vi "R vs T measurement.vi"() -> ()   [LabVIEW 2017]
uses:
  <vilib>/Utility/file.llb/Read Delimited Spreadsheet (DBL).vi
  <vilib>/Utility/file.llb/Write Delimited Spreadsheet (DBL).vi
  <instrlib>/Lake Shore 336/Lake Shore 336.lvlib
panel:
  in  "Tab Control":enum32{"Controlls", "Graphs", "Diagnositcs"}(tab)
  in  "Source Meter address":refnum<visa-resource-name>="GPIB1::29::INSTR"
  out "Measured Resistance (Ohms)":dbl format="%#_6p"
  in  "Resistance Range Lower Limit (2 Ohm)":dbl=2.0 format="%#_6p"
  in  "Resistance Range Upper Limit (2E+8 Ohm)":dbl=200000000.0 format="%#_6p"
  in  "Resistance NPLC (0.1)":dbl=0.1
  in  "Resistance Range (2 Ohm)":dbl=2.0
  in  "Resistance Auto Range (T: Enable)":bool=TRUE
  in  "file to save data (dialog if empty)":path
  in  "Temperature controller Addres":refnum<visa-resource-name>
  in  "Input (0:A)":u16(ring) items=["A", "B", "C", "D"]
  in  "Range (0:Off)":u16(ring) items=["Off", "Low (On)", "Medium", "High"]
  in  "Setpoint (0.00000)":dbl format="%.5f"
  in  "Enable Setpoint (F:Off)":bool
  out "Measured Resistance (K)":dbl format="%.6p"
  in  "Ramp Rate (0.0)":dbl format="%.1f"
  in  "Setpoint Ramping \nEnable (F: Off)":bool
  in  "Output's Control Loop (1:1)":u16(ring)=1 items=["1"=1, "2"=2]
  in  "Rate (D) (0.0 %)":dbl format="%.1f"
  in  "Reset (I) (20.0)":dbl=20.0 format="%.1f"
  in  "Gain (P) (50.0)":dbl=50.0 format="%.1f"
  in  "Mode (0:Off)":u16(ring) items=["Closed Loop PID", "Off", "Zone", "Open Loop"]
  in  "Max User Current (2.000)":dbl=2.0 format="%.3f"
  in  "Heater Out Display (1:Current)":u16(ring)=1 items=["Current"=1, "Power"=2]
  in  "Heater Resistance (1:25 Ohms)":u16(ring)=1 items=["50 Ohms"=2, "25 Ohms"=1]
  in  "Record Rate (ms)":u32=1000
  out "R T Graph":cluster{"all rows":dbl[], "all rows":dbl[]}(graph)
  in  "stop":bool
  in  "Error In":errorcluster
  # "Resistance vs Temperature Measurement"
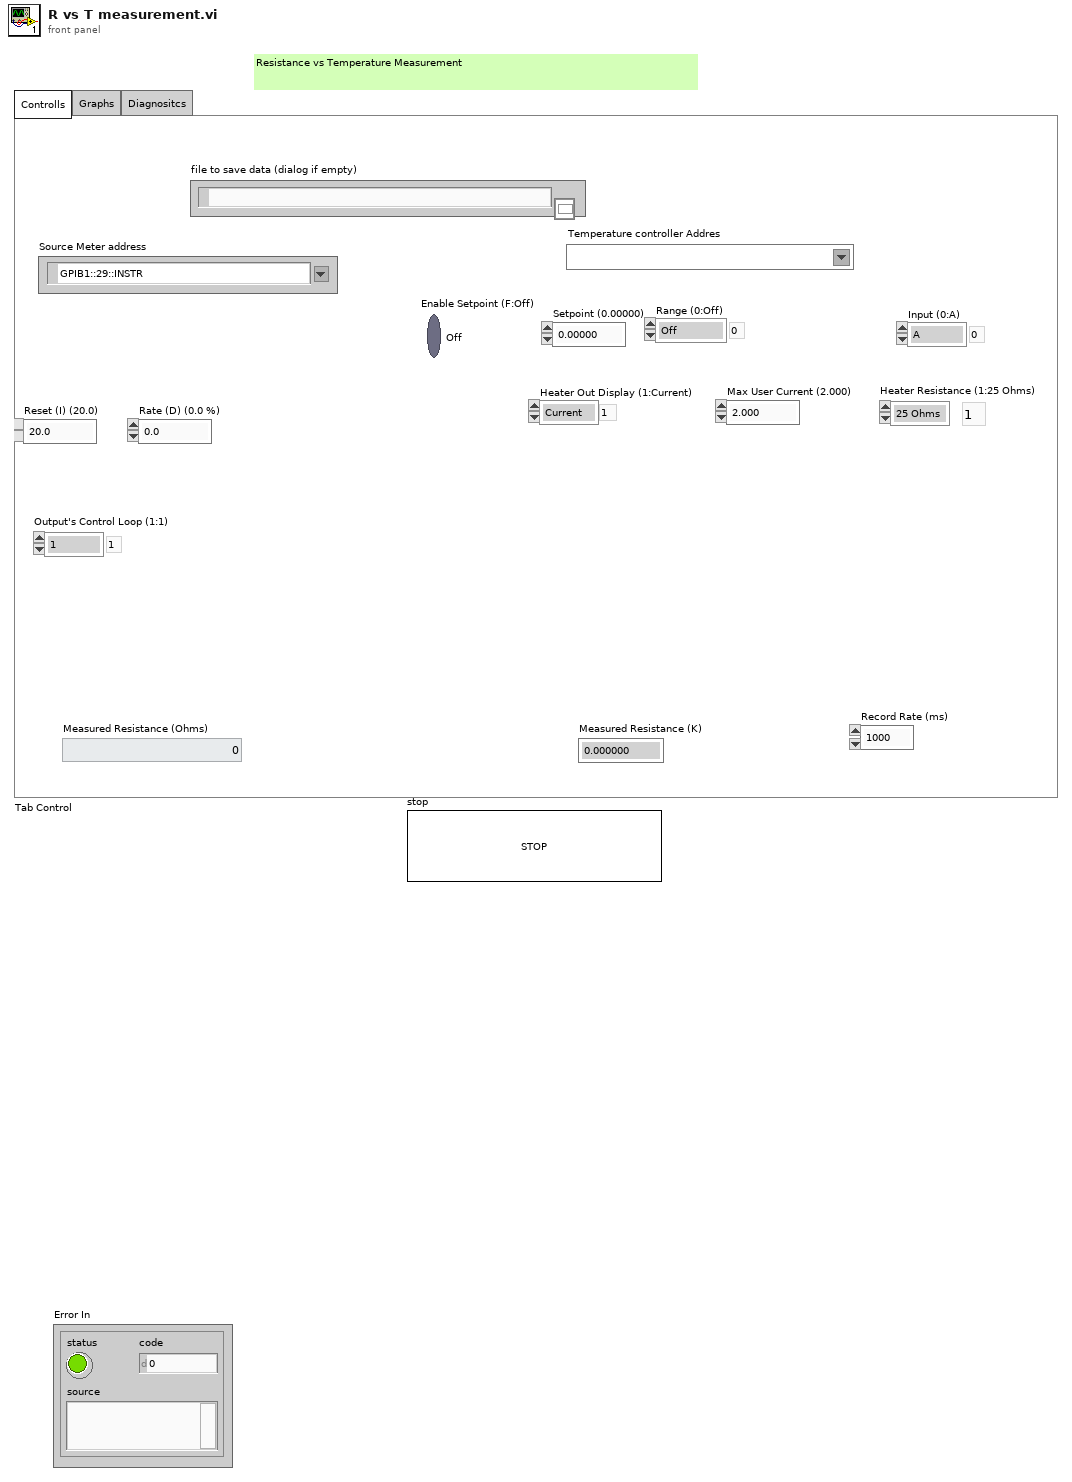
[diagram p1: front panel]
types:
  T1 = cluster{"Baud Rate":u32, "Parity":u16, "Data Bits":u16, "Stop Bits":u16, "Flow Control":u16}
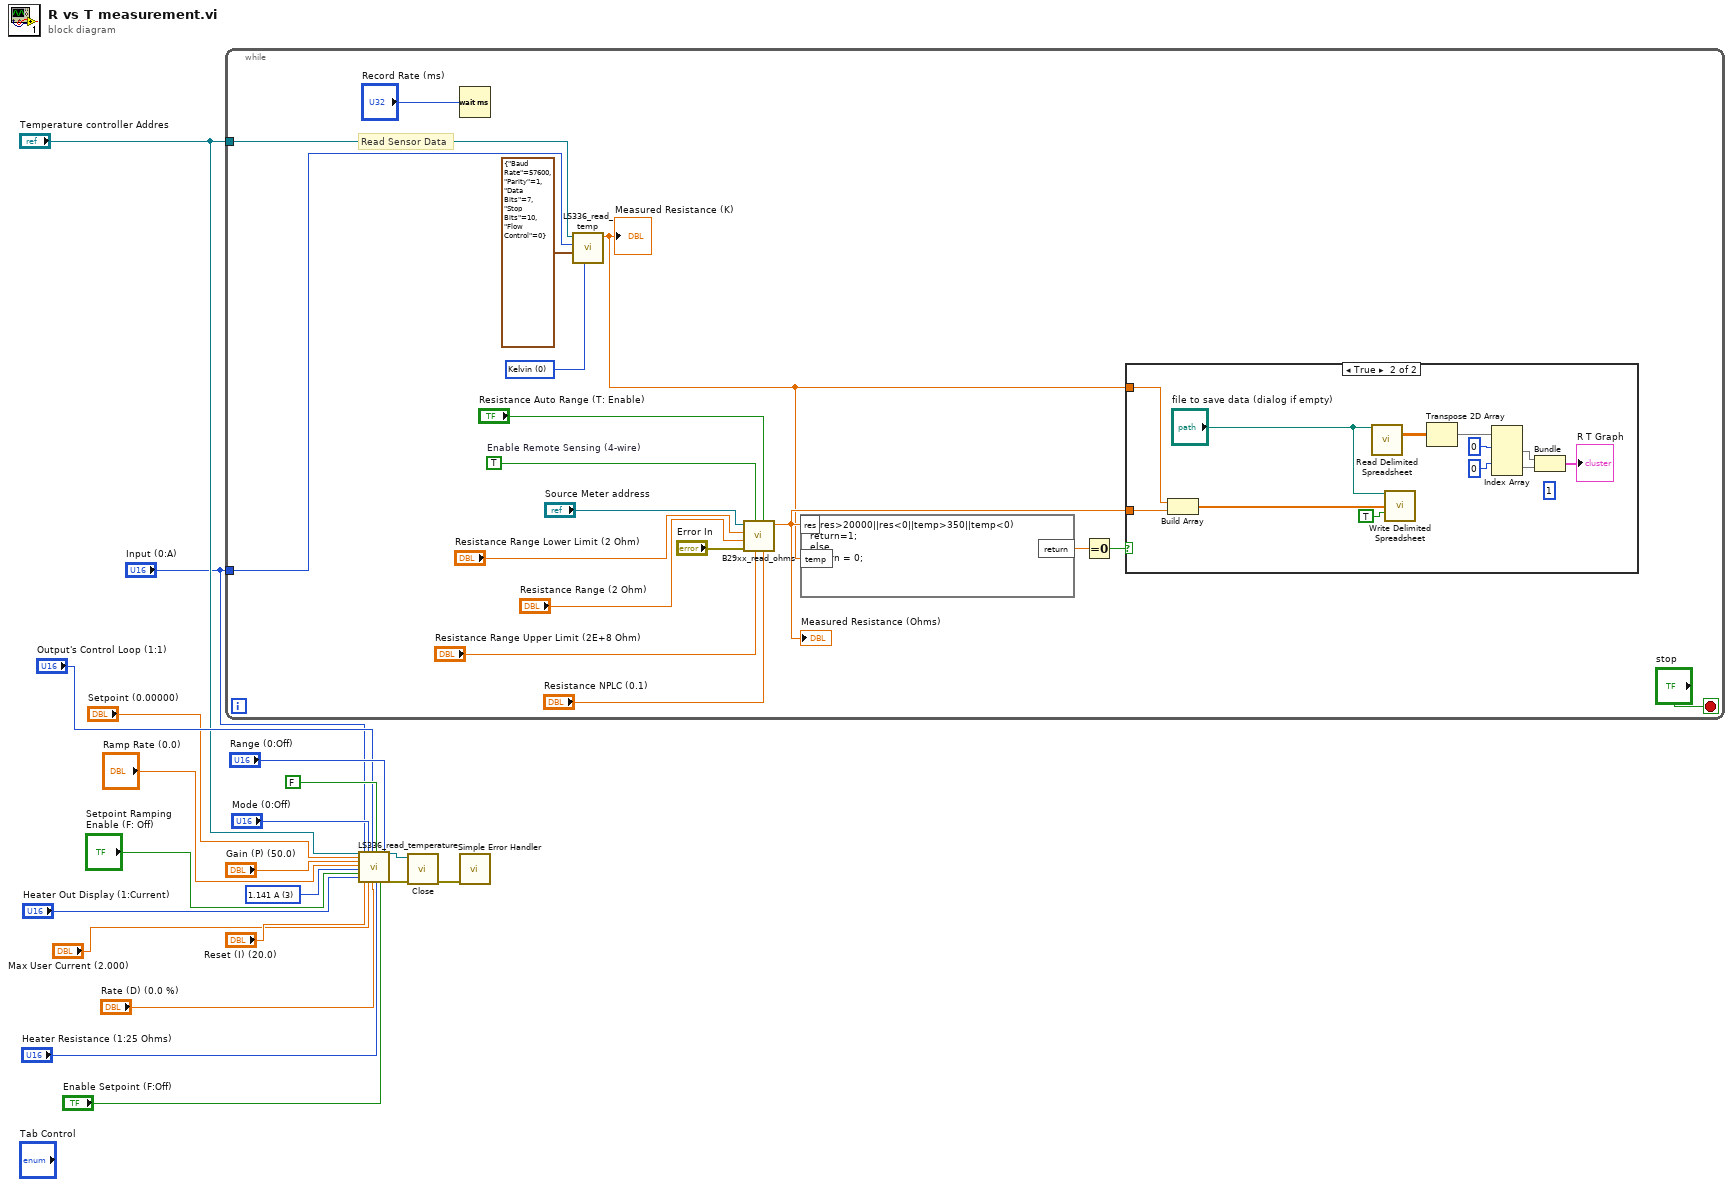
[diagram p0: block diagram]
diagram:
  w11 = u16 3 items=["User Specified", "0.707 A", "1.0 A", "1.141 A", "2.0 A"] ("Max Current (0:User Specified)")
  n1 = while {
    tunnel: "Temperature controller Addres" -> [w22]
    tunnel: "Input (0:A)" -> [w21]
    stop <- "stop" stop-if-true
    w24 = u16 0 items=["Kelvin", "Celsius", "Sensor Units"] ("Data Source (0:Kelvin)")
    w36 = TRUE  # Enable Remote Sensing (4-wire)
    # "Read Sensor Data"
    n2 = Wait (ms)(milliseconds to wait="Record Rate (ms)") -> ()  [unwired: 1 out]
    n3 = call "LS336_read_temp.vi"("Data Source (0:Kelvin)"=w24, "Serial Configuration"=T1 {"Baud Rate"=57600, "Parity"=1, "Data Bits"=7, "Stop Bits"=10, "Flow Control"=0}, "Input (0:A)"=w21, "VISA Refnum in"=w22) -> ("Sensor Data"=w23:dbl)  [unwired: 7 in]
    "Measured Resistance (K)" <- w23
    n4 = call "B29xx_read_ohms.vi"("Resistance NPLC (0.1)"="Resistance NPLC (0.1)", "Resistance Auto Range (T: Enable)"="Resistance Auto Range (T: Enable)", "Resistance Range Upper Limit (2E+8 Ohm)"="Resistance Range Upper Limit (2E+8 Ohm)", "Enable Remote Sensing (4-wire)"=w36, "error in (no error)"="Error In", "Resistance Range (2 Ohm)"="Resistance Range (2 Ohm)", "Resistance Range Lower Limit (2 Ohm)"="Resistance Range Lower Limit (2 Ohm)", "VISA Refnum in"="Source Meter address") -> ("Measurement Result"=w28:dbl)  [unwired: 2 in, 1 out]
    "Measured Resistance (Ohms)" <- w28
    n5 = formula code="if(res>20000||res<0||temp>350||temp<0)\nreturn=1;\nelse \nreturn = 0;"("res"=w28, "temp"=w23) -> ("return"=w30:dbl)
    n6 = Equal To 0?(x=w30) -> (x = 0?=w29:bool)
    n7 = case shown="True" w29 {
      tunnel: w28 -> [_ w48]
      tunnel: w23 -> [_ w43]
      frame False {
      }
      frame True {
        (unwired) 1 ("index (row)")
        n8 = Build Array(w43, w48) -> (w49:dbl[])
        n9 = call-poly <vilib>:"Read Delimited Spreadsheet.vi"("file path (dialog if empty)"="file to save data (dialog if empty)") -> ("all rows"=w41:dbl[][])  [unwired: 9 in, 5 out]
        n10 = call-poly <vilib>:"Write Delimited Spreadsheet.vi"("file path (dialog if empty)"="file to save data (dialog if empty)", "1D data"=w49, "append to file? (new file:F)"=TRUE) -> ()  [unwired: 11 in, 2 out]
        n11 = Transpose 2D Array(2D array=w41) -> (transposed array=w40:dbl[][])
        n12 = Index Array(array=w40, index (row) #1=0 ("index (row)"), index (row) #2=0 ("index (row)")) -> (element #1=w45:dbl[], element #2=w46:dbl[])  [unwired: 2 in]
        n13 = Bundle(w45, w46) -> (→"R T Graph":cluster{dbl[], dbl[]})  [unwired: 1 in]
      }
    }
  }
  n14 = call "LS336_read_temperature.vi"("VISA Refnum in"="Temperature controller Addres", "Setpoint (0.00000)"="Setpoint (0.00000)", "Gain (P) (50.0)"="Gain (P) (50.0)", "Ramp Rate (0.0)"="Ramp Rate (0.0)", "Max Current (0:User Specified)"=w11, "Setpoint Ramping \nEnable (F: Off)"="Setpoint Ramping \nEnable (F: Off)", "Heater Out Display (1:Current)"="Heater Out Display (1:Current)", "Input (0:None)"="Input (0:A)", "Reset (I) (20.0)"="Reset (I) (20.0)", "Mode (0:Off)"="Mode (0:Off)", "Max User Current (2.000)"="Max User Current (2.000)", "Output's Control Loop (1:1)"="Output's Control Loop (1:1)", "Rate (D) (0.0 %)"="Rate (D) (0.0 %)", "Power Up Enable (F: Off)"=FALSE, "Heater Resistance (1:25 Ohms)"="Heater Resistance (1:25 Ohms)", "Enable Setpoint (F:Off)"="Enable Setpoint (F:Off)", "Range (0:Off)"="Range (0:Off)") -> ("VISA Refnum out"=w19:refnum<visa-resource-name>, "error out"=w20:errorcluster)  [unwired: 9 in]
  n15 = call <instrlib>:"Close.vi"("error in (no error)"=w20, "VISA resource name"=w19) -> ("error out"=w7:errorcluster)  [unwired: 9 in]
  n16 = call <vilib>:"Simple Error Handler.vi"("error in (no error)"=w7) -> ()  [unwired: 4 in, 5 out]
